vi "Test.vi"() -> ()   [LabVIEW 2013]
panel:
  out "controlState":dbl[](array[numeric])=[-6.74]
  in  "Code":string="x=plantState[1];\ncontrolState[0]=-x;\nfor (i=0; i<1000000 ; i++);"
  in  "plantState":dbl[](array[numeric])=[1.0, 6.74]
  out "evals1":i32=713
  out "T1":u32(graph)=320
  in  "stop":bool=TRUE
  out "error out":errorcluster
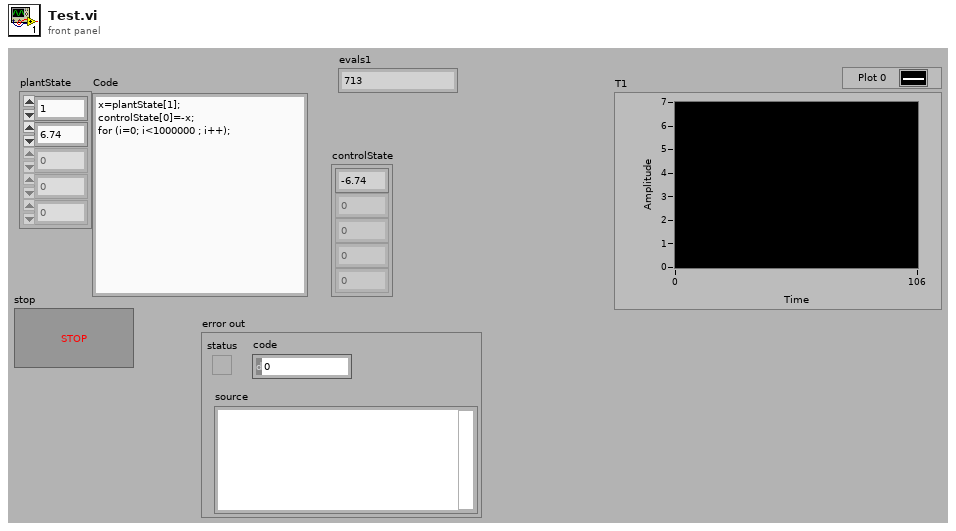
[diagram p1: front panel]
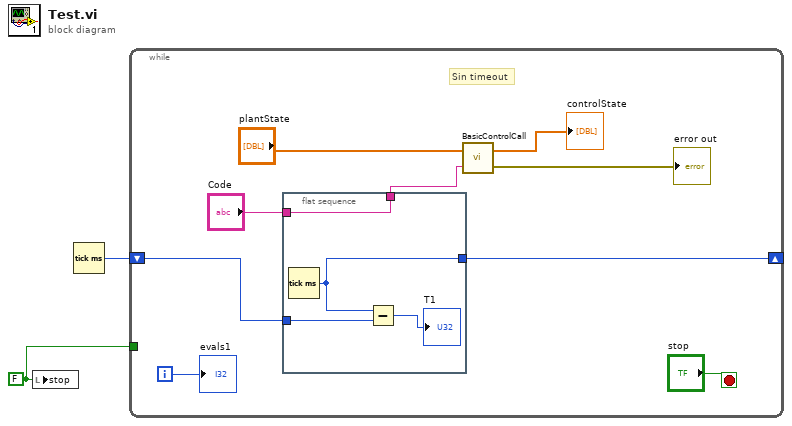
[diagram p0: block diagram]
diagram:
  w2 = FALSE ("stop")
  n1 = local write "stop"(w2) -> ()
  n2 = Tick Count (ms)() -> (millisecond timer value=w1:u32)
  n3 = while {
    shift-right: [w7] -> _
    shift-left: w1 -> [w6]
    tunnel: w2 -> [_]
    i -> [w10]
    stop <- "stop" stop-if-true
    # "Sin timeout"
    n4 = flat-sequence {
      tunnel: [w15] -> w7
      tunnel: w6 -> [w14]
      tunnel: [w12] -> w4
      tunnel: "Code" -> [w12]
      frame #0 {
        n5 = Tick Count (ms)() -> (millisecond timer value=w15:u32)
        n6 = Subtract(x=w15, y=w14) -> (x-y=→"T1":u32)
      }
    }
    n7 = call "BasicControlCall.vi"("Code"=w4, "plantState"="plantState") -> ("error"=→"error out":errorcluster, "controlState"=→"controlState":dbl[])
    "evals1" <- w10
  }
